vi "Get FPGA uService ID.vi"(6 "error in":errorcluster, 8 "FPGA Name":string, 9 "FPGA Interface":refnum<class "FPGA Interface.lvclass">) -> (0 "error out":errorcluster, 1 "uService ID":string, 2 "uService Class Name":string)   [LabVIEW 2026, in "TALOS.lvlib" / "Interfaces.lvlib" / "FPGA Interface.lvclass"]
uses:
  FPGA Interface.lvclass
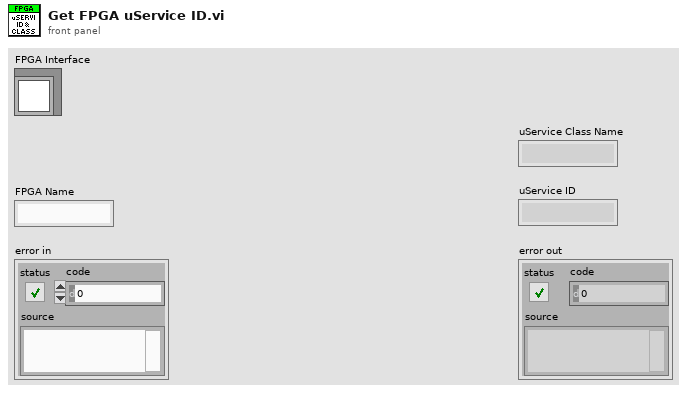
[diagram p1: front panel]
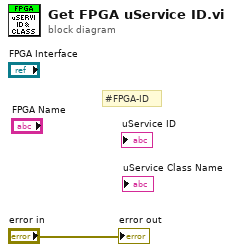
[diagram p0: block diagram]
diagram:
  # "#FPGA-ID"
  "error out" <- "error in"
